vi "Audio_Transformation_Setted_Frequency_v005.vi"() -> ()   [LabVIEW 2019]
uses:
  <vilib>/addons/_Advanced Signal Processing/NI_AdvSigProcTFA.lvlib
  <vilib>/sound2/lvsound2.llb/Sound Data Format.ctl
  <vilib>/sound2/lvsound2.llb/Sound Input Read (DBL).vi
  <vilib>/addons/Time Frequency Analysis/Transform.llb/TFA Online Gabor Transform (Real).vi
panel:
  out "u(t)":T1(graph)
  out "V(t)":T1(graph)
  out "Noise Speech":dbl[](graph)
  in  "Address selector":i32[](array[numeric])
  in  "Neuron Type":T2(ring)
  out "max index(es)":i32
  out "max value":dbl
  out "Waveform Graph":dbl[](graph)
  out "Magnitude of Gabor Coefficients":dbl[][](graph)
  in  "Stop":bool
  # "Step two : Graph of the amplitude of the Gabor coefficient of the different bins"
  # "Step three : Spike Response of the neurons"
  # "Step one: Sound recorded from the computer"
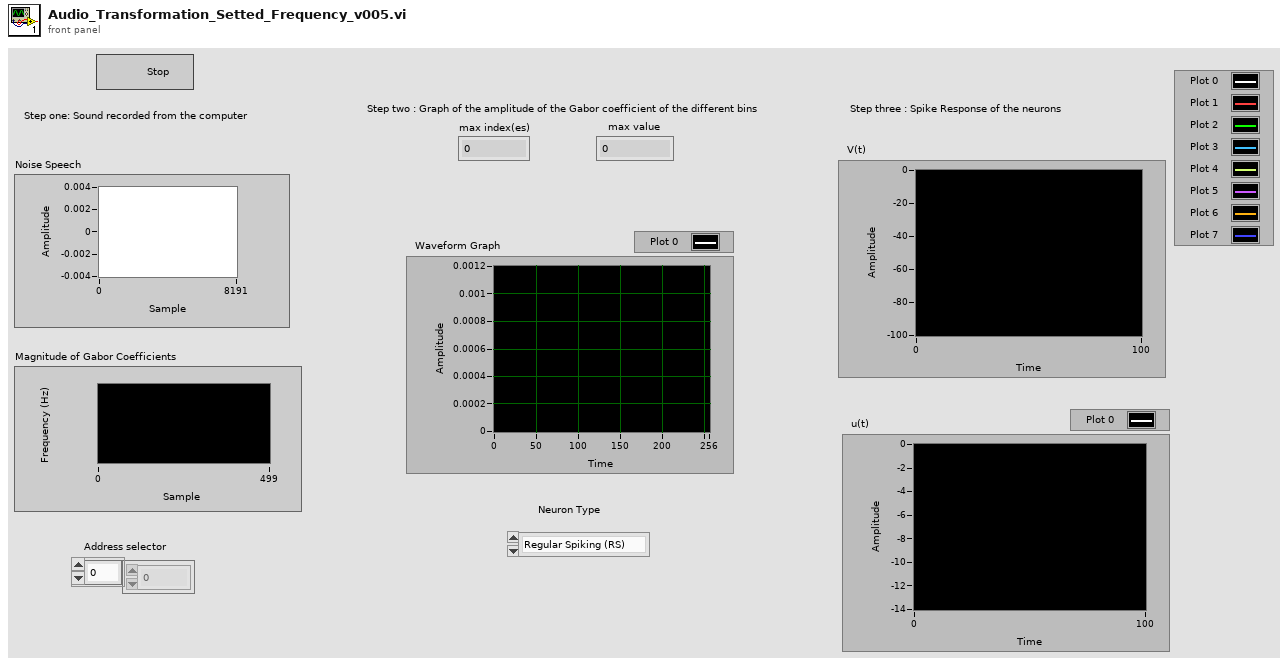
[diagram p1: front panel]
types:
  T1 = cluster{"[0]":dbl, "[1]":dbl, "[2]":dbl, "[3]":dbl, "[4]":dbl, "[5]":dbl, "[6]":dbl, "[7]":dbl}
  T2 = enum16{"Regular Spiking (RS)", "Intrinsically Bursting (IB)", "Chattering (CH)", "Fast Spiking (FS)", "Thalamo-Cortical 1 (TC1)", "Thalamo-Cortical 2 (TC2)", "Resonator (RZ)", "Low-Threshold Spiking (LTS)"}
  T3 = typedef "Sound Data Format.ctl" = cluster{"sample rate (S/s)":dbl, "number of channels":i32, "bits per sample":i32}
  T4 = typedef "Sound Input Task ID.ctl" = u32
  T5 = cluster{"analysis window":dbl[], "dM (time steps)":i32, "N (frequency bins)":i32}
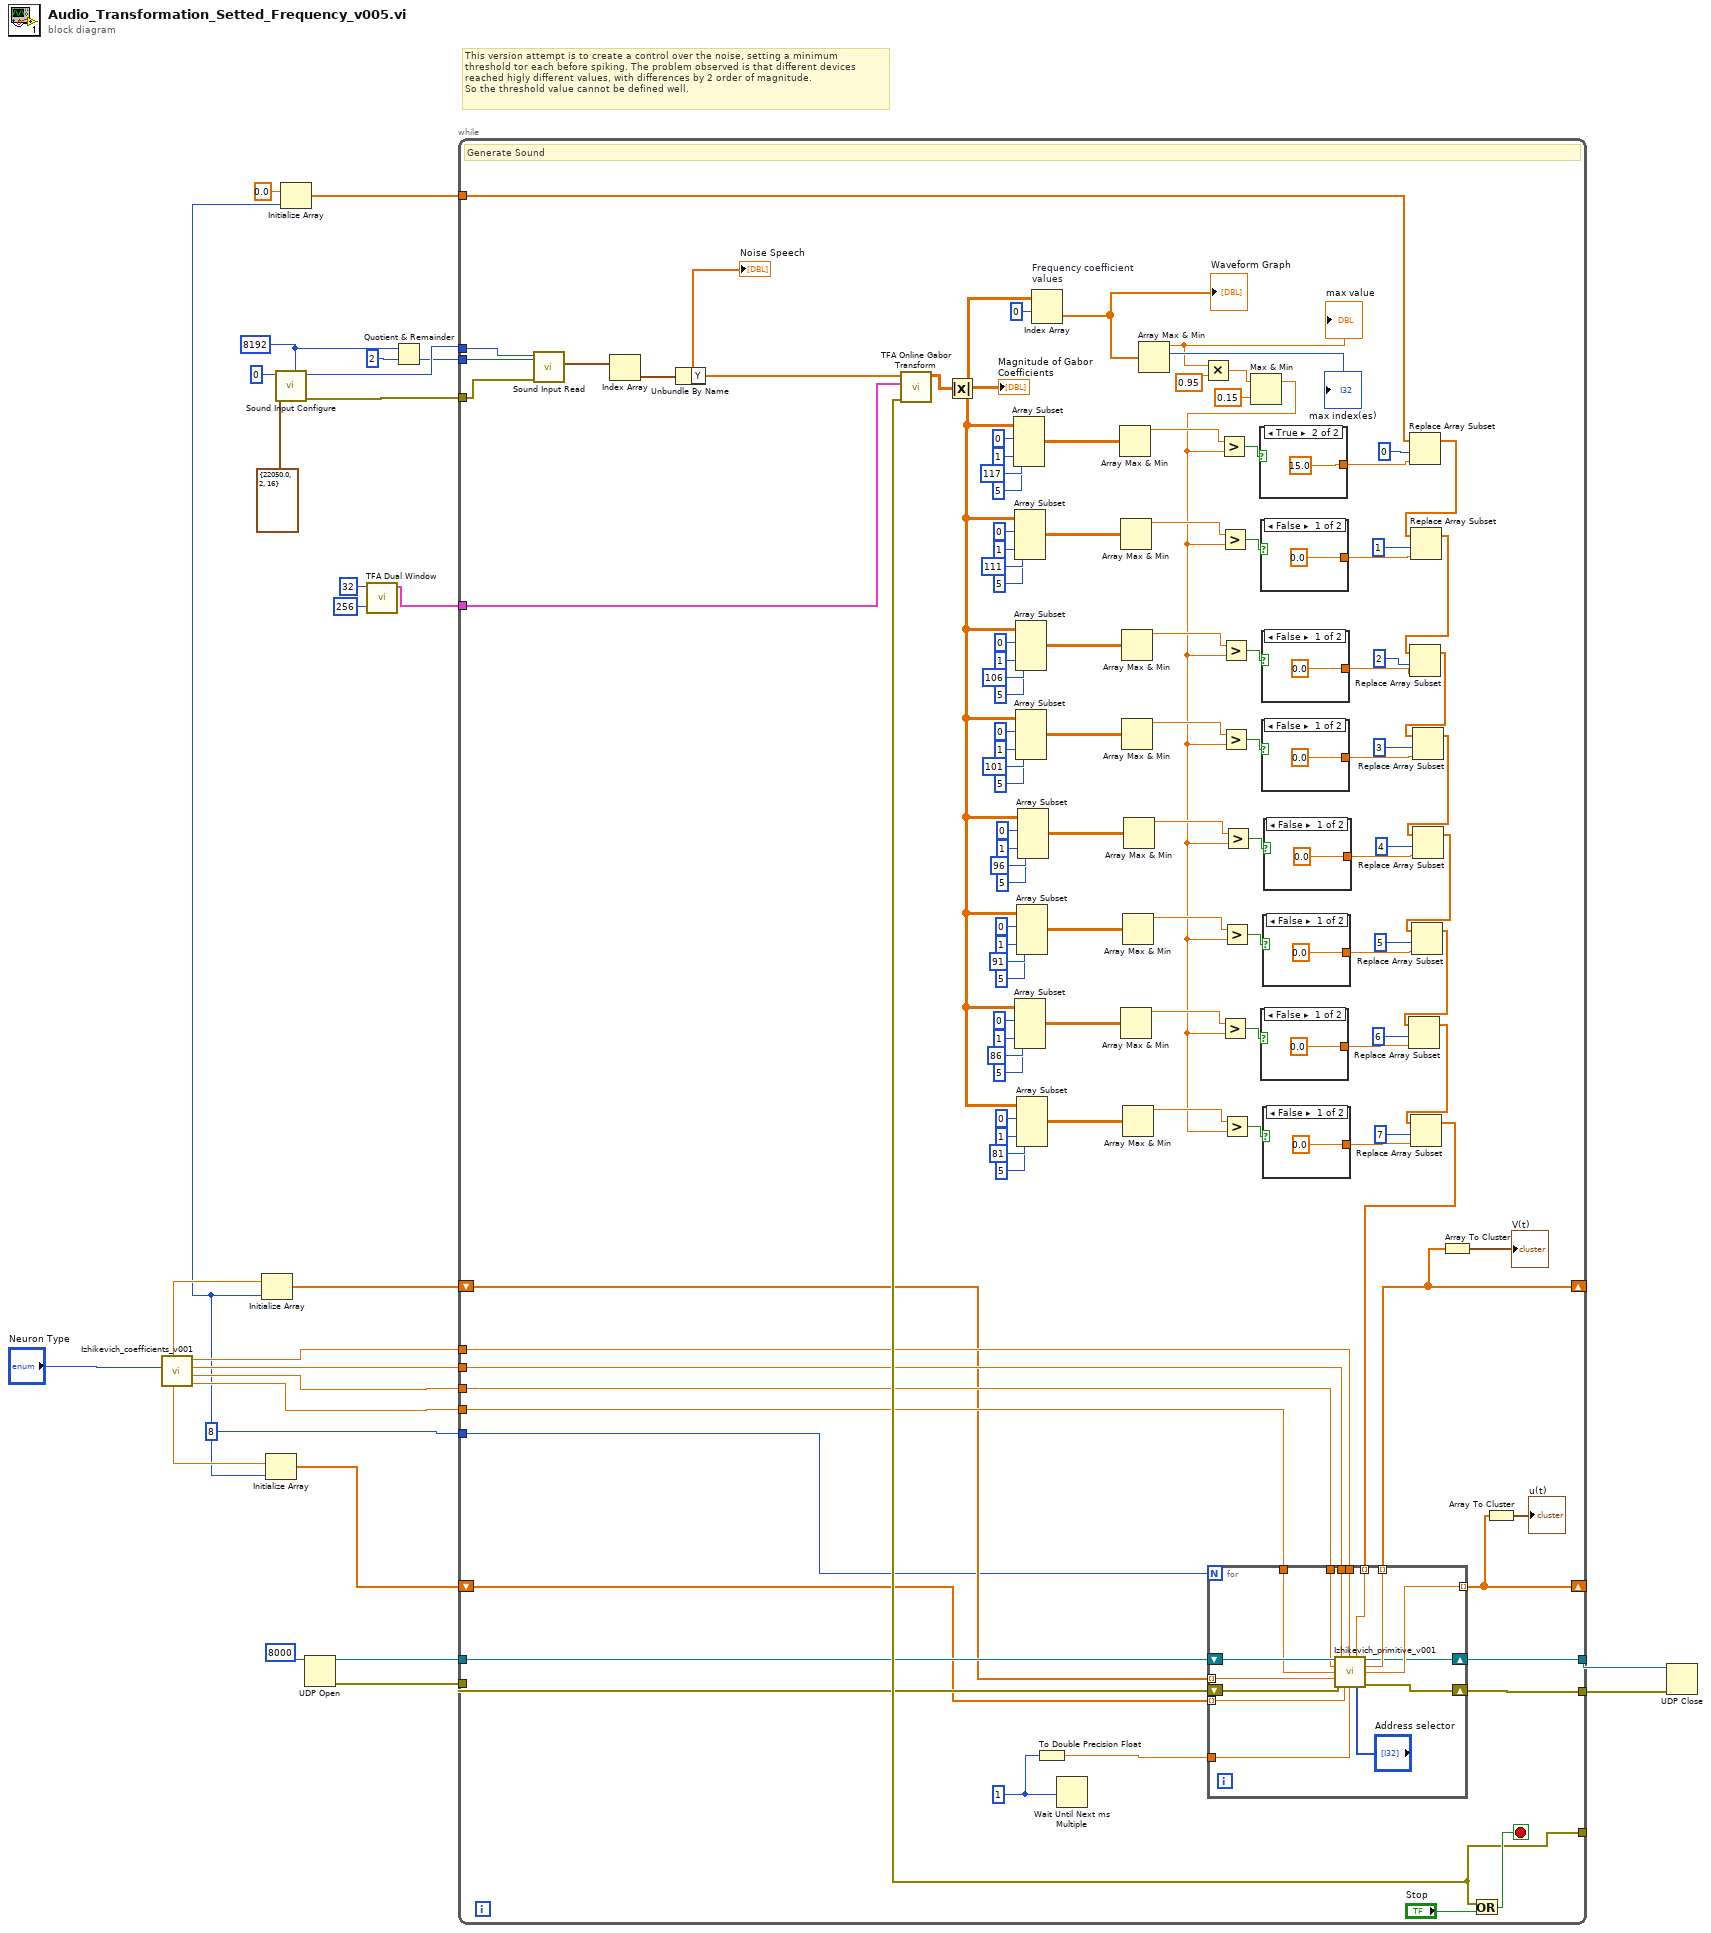
[diagram p0: block diagram]
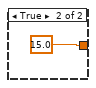
[diagram p2: hidden frame]
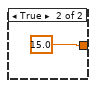
[diagram p3: hidden frame]
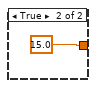
[diagram p4: hidden frame]
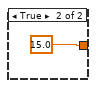
[diagram p5: hidden frame]
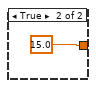
[diagram p6: hidden frame]
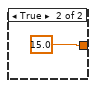
[diagram p7: hidden frame]
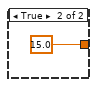
[diagram p8: hidden frame]
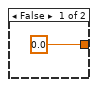
[diagram p9: hidden frame]
diagram:
  w3 = 8
  w12 = 8192 ("number of samples/ch")
  # "This version attempt is to create a control over the noise, setting a minimum\nthreshold tor each before spiking. The problem observed is that different devices\nreached higly different values, with differences by 2 order of magnitude.\nSo the threshold value cannot be defined well."
  n1 = call "Izhikevich_coefficients_v001.vi"("Neuron Type"="Neuron Type") -> ("d"=w20:dbl, "c"=w21:dbl, "b"=w22:dbl, "a"=w23:dbl, "u0"=w5:dbl, "v0"=w7:dbl)  [unwired: 3 in]
  n2 = Initialize Array(w7, w3) -> (w6:dbl[])
  n3 = Initialize Array(w5, w3) -> (w4:dbl[])
  n4 = call <vilib>:"Sound Input Configure.vi"("number of samples/ch"=w12, "sound format"=T3 {"sample rate (S/s)"=22050.0, "number of channels"=2, "bits per sample"=16}, "device ID"=u32 0) -> ("error out"=w9:errorcluster, "task ID"=w10:T4)  [unwired: 7 in]
  n5 = Initialize Array(0.0 ("element"), w3) -> (w1:dbl[])
  n6 = UDP Open(11:u16 8000 ("port")) -> (port=w18:refnum<k16>, 0:w17:errorcluster)  [unwired: 4 in, 1 out]
  n7 = call <vilib>:"TFA Dual Window.vi"("N (frequency bins)"=256, "dM (time steps)"=32) -> ("analysis info"=w25:T5)  [unwired: 7 in, 2 out]
  n8 = Quotient & Remainder(x=w12, y=2) -> (floor(x/y)=w8:i32)  [unwired: 1 out]
  n9 = while {
    tunnel: [w138] -> _
    tunnel: w25 -> [w143]
    shift-right: [w34] -> _
    shift-left: w6 -> [w127]
    shift-right: [w32] -> _
    shift-left: w4 -> [w126]
    tunnel: w23 -> [w137]
    tunnel: w22 -> [w136]
    tunnel: w21 -> [w134]
    tunnel: w20 -> [w133]
    tunnel: w18 -> [w135]
    tunnel: w17 -> [w132]
    tunnel: [w129] -> w16
    tunnel: [w128] -> w15
    tunnel: w10 -> [w124]
    tunnel: w9 -> [w123]
    tunnel: w8 -> [w125]
    tunnel: w3 -> [w119]
    tunnel: w1 -> [w90]
    stop <- w144 stop-if-true
    w131 = u32 1 ("millisecond multiple")
    # "Generate Sound"
    n10 = call-poly <vilib>:"Sound Input Read.vi"("number of samples/ch"=w125, "error in (no error)"=w123, "task ID"=w124) -> ("data"=w121:waveform(dbl)[])  [unwired: 6 in, 2 out]
    n11 = Index Array(array=w121) -> (element=w122:waveform(dbl))  [unwired: 1 in]
    n12 = Unbundle By Name(w122) -> ("Y"=w120:dbl[])
    "Noise Speech" <- w120
    n13 = call-poly <vilib>:"TFA Online Gabor Transform.vi"("transform info"=w143, "signal"=w120) -> ("error out"=w138:errorcluster, "Gabor coef"=w142:cdb[][])  [unwired: 7 in, 1 out]
    n14 = Absolute Value(x=w142) -> (abs(x)=w38:dbl[][])
    "Magnitude of Gabor Coefficients" <- w38
    n15 = Array Subset(array=w38, index (row)=0 ("index"), length (row)=1 ("length"), index (col)=117 ("index"), length (col)=5 ("length")) -> (w114:dbl[][])
    n16 = Array Subset(array=w38, index (row)=0 ("index"), length (row)=1 ("length"), index (col)=111 ("index"), length (col)=5 ("length")) -> (w106:dbl[][])
    n17 = Array Subset(array=w38, index (row)=0 ("index"), length (row)=1 ("length"), index (col)=86 ("index"), length (col)=5 ("length")) -> (w53:dbl[][])
    n18 = Array Subset(array=w38, index (row)=0 ("index"), length (row)=1 ("length"), index (col)=106 ("index"), length (col)=5 ("length")) -> (w95:dbl[][])
    n19 = Array Subset(array=w38, index (row)=0 ("index"), length (row)=1 ("length"), index (col)=101 ("index"), length (col)=5 ("length")) -> (w83:dbl[][])
    n20 = Array Subset(array=w38, index (row)=0 ("index"), length (row)=1 ("length"), index (col)=91 ("index"), length (col)=5 ("length")) -> (w63:dbl[][])
    n21 = Array Subset(array=w38, index (row)=0 ("index"), length (row)=1 ("length"), index (col)=81 ("index"), length (col)=5 ("length")) -> (w43:dbl[][])
    n22 = Array Subset(array=w38, index (row)=0 ("index"), length (row)=1 ("length"), index (col)=96 ("index"), length (col)=5 ("length")) -> (w73:dbl[][])
    n23 = Index Array "Frequency coefficient \nvalues"(array=w38, index (row)=0) -> (element=w140:dbl[])  [unwired: 1 in]
    "Waveform Graph" <- w140
    n24 = To Double Precision Float(number=w131) -> (double precision float=w130:dbl)
    n25 = Wait Until Next ms Multiple(millisecond multiple=w131) -> ()  [unwired: 1 out]
    n26 = Array Max & Min(array=w114) -> (max value=w112:dbl)  [unwired: 3 out]
    n27 = Array Max & Min(array=w106) -> (max value=w105:dbl)  [unwired: 3 out]
    n28 = Array Max & Min(array=w53) -> (max value=w52:dbl)  [unwired: 3 out]
    n29 = Array Max & Min(array=w95) -> (max value=w94:dbl)  [unwired: 3 out]
    n30 = Array Max & Min(array=w83) -> (max value=w82:dbl)  [unwired: 3 out]
    n31 = Array Max & Min(array=w63) -> (max value=w62:dbl)  [unwired: 3 out]
    n32 = Array Max & Min(array=w43) -> (max value=w42:dbl)  [unwired: 3 out]
    n33 = Array Max & Min(array=w73) -> (max value=w72:dbl)  [unwired: 3 out]
    n34 = Array Max & Min(array=w140) -> (max value=w113:dbl, max index (indices)=→"max index(es)":i32)  [unwired: 2 out]
    "max value" <- w113
    n35 = Multiply(x=w113, y=0.95) -> (x*y=w30:dbl)
    n36 = Max & Min(x=w30, y=0.15) -> (max(x,y)=w28:dbl)  [unwired: 1 out]
    n37 = Greater?(x=w112, y=w28) -> (0:w111:bool)
    n38 = Greater?(x=w105, y=w28) -> (0:w104:bool)
    n39 = Greater?(x=w52, y=w28) -> (0:w51:bool)
    n40 = Greater?(x=w94, y=w28) -> (0:w93:bool)
    n41 = Greater?(x=w82, y=w28) -> (0:w81:bool)
    n42 = Greater?(x=w62, y=w28) -> (0:w61:bool)
    n43 = Greater?(x=w42, y=w28) -> (0:w41:bool)
    n44 = Greater?(x=w72, y=w28) -> (0:w71:bool)
    n45 = case shown="True" w111 {
      tunnel: [0.0 15.0] -> w103
      frame False {
      }
      frame True {
      }
    }
    n46 = case shown="False" w104 {
      tunnel: [0.0 15.0] -> w100
      frame False {
      }
      frame True {
      }
    }
    n47 = case shown="False" w51 {
      tunnel: [0.0 15.0] -> w49
      frame False {
      }
      frame True {
      }
    }
    n48 = case shown="False" w93 {
      tunnel: [0.0 15.0] -> w91
      frame False {
      }
      frame True {
      }
    }
    n49 = case shown="False" w81 {
      tunnel: [0.0 15.0] -> w79
      frame False {
      }
      frame True {
      }
    }
    n50 = case shown="False" w61 {
      tunnel: [0.0 15.0] -> w59
      frame False {
      }
      frame True {
      }
    }
    n51 = case shown="False" w41 {
      tunnel: [0.0 15.0] -> w39
      frame False {
      }
      frame True {
      }
    }
    n52 = case shown="False" w71 {
      tunnel: [0.0 15.0] -> w69
      frame False {
      }
      frame True {
      }
    }
    n53 = Replace Array Subset(array=w90, new element=w103, index=0) -> (w89:dbl[])
    n54 = Replace Array Subset(array=w89, new element=w100, index=1) -> (w88:dbl[])
    n55 = Replace Array Subset(array=w88, new element=w91, index=2) -> (w78:dbl[])
    n56 = Replace Array Subset(array=w78, new element=w79, index=3) -> (w68:dbl[])
    n57 = Replace Array Subset(array=w68, new element=w69, index=4) -> (w58:dbl[])
    n58 = Replace Array Subset(array=w58, new element=w59, index=5) -> (w48:dbl[])
    n59 = Replace Array Subset(array=w48, new element=w49, index=6) -> (w36:dbl[])
    n60 = Replace Array Subset(array=w36, new element=w39, index=7) -> (w35:dbl[])
    n61 = for {
      N: w119 -> [_]
      tunnel: w137 -> [w176]
      tunnel: w136 -> [w175]
      tunnel: w134 -> [w173]
      tunnel: w133 -> [w172]
      tunnel: w130 -> [w169]
      tunnel: [w168] -> w34 mode=indexing
      tunnel: [w167] -> w32 mode=indexing
      tunnel: w127 -> [w164] mode=indexing
      tunnel: w126 -> [w163] mode=indexing
      shift-right: [w165] -> w128
      shift-left: w135 -> [w174]
      shift-right: [w166] -> w129
      shift-left: w132 -> [w171]
      tunnel: w35 -> [w162] mode=indexing
      n62 = call "Izhikevich_primitive_v001.vi"("UDP Network Connection in"=w174, "b"=w175, "a"=w176, "I"=w162, "c"=w173, "d"=w172, "v(t)"=w164, "error in (no error)"=w171, "u(t)"=w163, "Numeric"=w169, "Address selector"="Address selector") -> ("UDP Network Connection out"=w165:refnum<k16>, "v(t+dt)"=w168:dbl, "u(t+dt)"=w167:dbl, "error out"=w166:errorcluster)  [unwired: 1 in]
    }
    n63 = Array To Cluster(array=w34) -> (cluster=→"V(t)":T1)
    n64 = Or(x=w138, y="Stop") -> (x .or. y?=w144:bool)
    n65 = Array To Cluster(array=w32) -> (cluster=→"u(t)":T1)
  }
  n66 = UDP Close(connection ID=w15, 8:w16) -> ()  [unwired: 2 out]
